vi "HFRR ADV v032 new software.vi"() -> ()   [LabVIEW 2025] (continued)
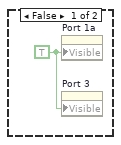
[diagram p5: hidden frame]
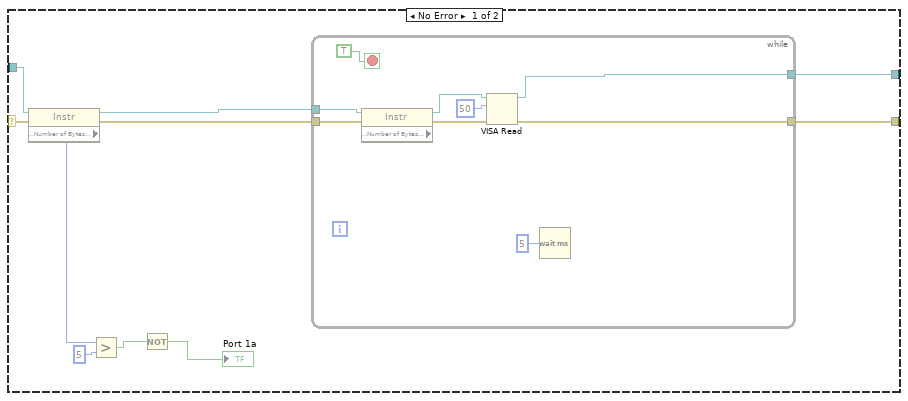
[diagram p6: hidden frame]
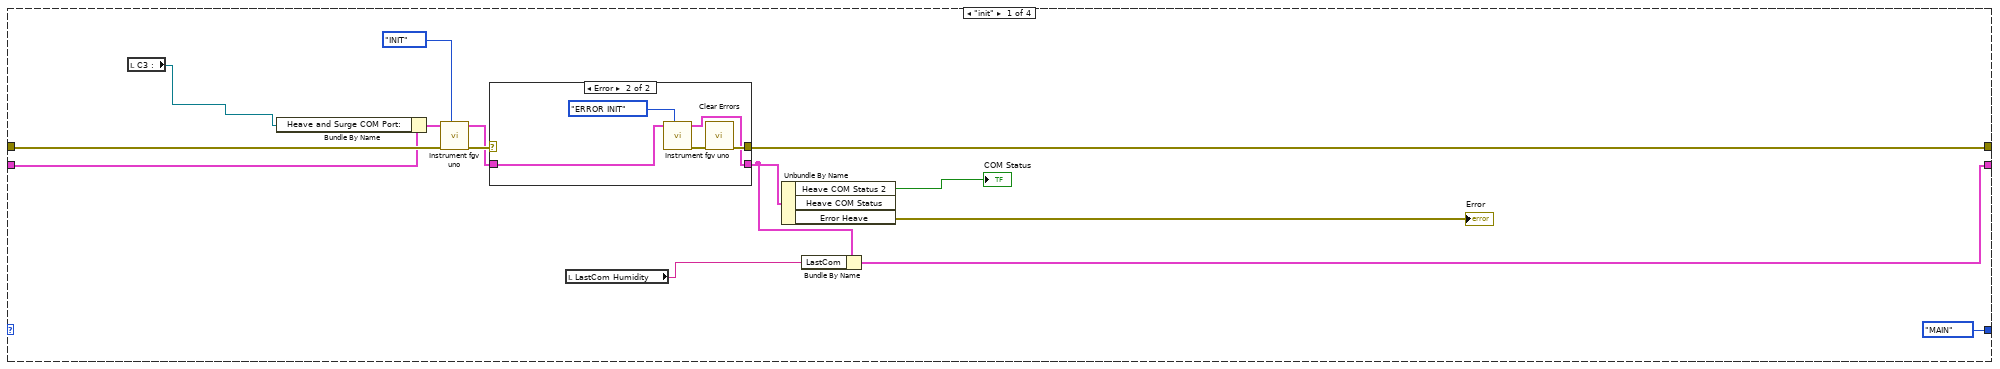
[diagram p8: hidden frame]
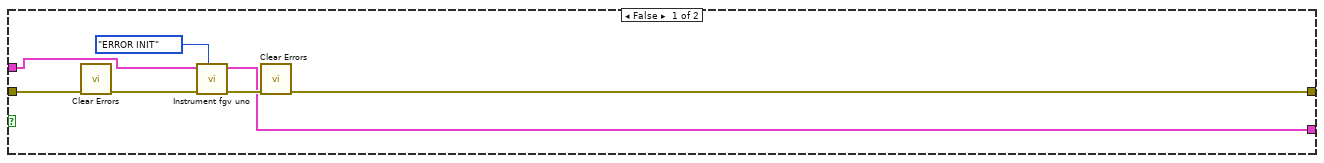
[diagram p10: hidden frame]
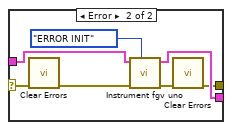
[diagram p12: hidden frame]
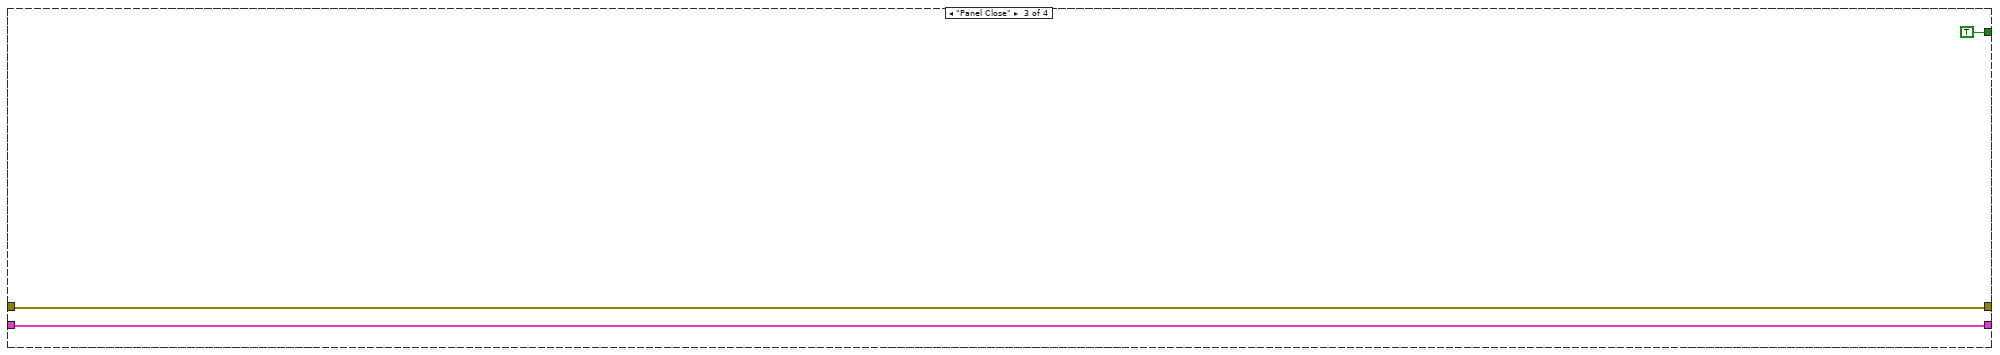
[diagram p14: hidden frame]
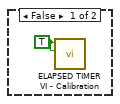
[diagram p18: hidden frame]
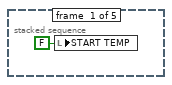
[diagram p20: hidden frame]
    shift-left: T20 {"Read Uno"="", "Bytes at Heave Port"=0.0, "UNO COM Port:"="COM9", "UNO COM Port: 2"="COM7", "Residual Due"="", "UNO COM Status 2"=TRUE, "UNO COM Status"=TRUE, "Port 2"=TRUE, "Sway PPR"=6400.0, "Surge PPR"=6400.0, "Heave PPR"=6400.0, "Sway Pitch"=2.0, "Surge Pitch"=3.0, "Heave Pitch"=4.0, "Sway Pulses/mm"=320.0, "Surge Pulses/mm"=1600.0, "Heave Pulses/mm"=1600.0, "inner loop"=0.0, "Read Heave and Surge 2"="", "String 36"="", "Write S"=FALSE, "WriteCC1"=[""], "Heave COM Loop"=0, "LastCom"="", "EXIT"=FALSE, "Error Heave"={"status"=TRUE, "code"=-1073807343, "source"=""}} -> [w4388]
    shift-right: [w4386] -> _
    shift-left: enum16{"init", "MAIN", "Panel Close"}."init" -> [w4387]
    stop <- w4390 stop-if-true
    # "UNO CODE LOGIC"
    n3353 = case shown="\"MAIN\"" w4387 {
      tunnel: w4392 -> [w4406 w4425 w4481 w4483]
      tunnel: [w4401 w4430 w4481 w4483] -> w4391
      tunnel: [_ _ TRUE _] -> w4390
      tunnel: [w4397 w4428 w4479 w4482] -> w4389
      tunnel: w4388 -> [w4403 w4424 w4479 w4482]
      tunnel: [enum16{"init", "MAIN", "Panel Close"}."MAIN" w4419 _ _] -> w4386
      frame "init" {
        n3354 = local read "Com Port 1"() -> (w4393:refnum<visa-resource-name>)
        n3355 = Bundle By Name(cluster=w4403, "UNO COM Port:"=w4393) -> (w4402:T20)
        n3356 = call "Instrument fgv.vi"("Enum"=T31."INIT", "error in (no error) 2"=w4406, "INPUT"=w4402) -> ("error"=w4404:errorcluster, "output"=w4400:T18)  [unwired: 6 in, 1 out]
        n3357 = case shown="Error" w4404 {
          selector: w4404 -> [w4408 _]
          tunnel: [w4408 w4412] -> w4401
          tunnel: w4400 -> [w4407 w4410]
          tunnel: [w4407 w4409] -> w4398
          frame No Error {
          }
          frame Error {
            n3358 = call "Instrument fgv.vi"("Enum"=T31."ERROR INIT", "INPUT"=w4410) -> ("error"=w4413:errorcluster, "output"=w4409:T18)  [unwired: 7 in, 1 out]
            n3359 = call <vilib>:"Clear Errors.vi"("error in (no error)"=w4413) -> ("error out"=w4412:errorcluster)  [unwired: 5 in, 1 out]
          }
        }
        n3360 = local read "LastCom UNO"() -> (w4395:string)
        n3361 = Unbundle By Name(w4398) -> ("Heave COM Status 2"=→"Instrument Status":bool, "Error Heave"=→"Error  2":errorcluster)  [unwired: 1 out]
        n3362 = Bundle By Name(cluster=w4398, "LastCom"=w4395) -> (w4397:T18)
      }
      frame "MAIN" {
        n3363 = Unbundle By Name(w4424) -> ("UNO COM Port: 2"=w4414:refnum<visa-resource-name>)
        n3364 = local read "Com Port 1"() -> (w4415:refnum<visa-resource-name>)
        n3365 = local write "COM Port UNO :"(w4414) -> ()
        n3366 = Equal?(x=w4414, y=w4415) -> (x = y?=w4431:bool)
        n3367 = Bundle By Name(cluster=w4424, "UNO COM Port:"=w4415) -> (w4423:T20)
        n3368 = case shown="True" w4431 {
          tunnel: [w4435 w4452] -> w4430
          tunnel: w4425 -> [w4436 w4458]
          tunnel: w4423 -> [w4434 w4456]
          tunnel: [w4433 w4451] -> w4428
          frame False {
            n3369 = call <vilib>:"Clear Errors.vi"("error in (no error)"=w4436) -> ("error out"=w4432:errorcluster)  [unwired: 5 in, 1 out]
            n3370 = call "Instrument fgv.vi"("Enum"=T31."ERROR INIT", "error in (no error) 2"=w4432, "INPUT"=w4434) -> ("error"=w4438:errorcluster, "output"=w4433:T18)  [unwired: 6 in, 1 out]
            n3371 = call <vilib>:"Clear Errors.vi"("error in (no error)"=w4438) -> ("error out"=w4435:errorcluster)  [unwired: 5 in, 1 out]
          }
          frame True {
            n3372 = call "Instrument fgv.vi"("Enum"=T31."READ", "error in (no error) 2"=w4458, "INPUT"=w4456) -> ("error"=w4457:errorcluster, "output"=w4450:T18)  [unwired: 6 in, 1 out]
            n3373 = Bundle By Name(cluster=w4450, "String 36"="WRITE UNO") -> (w4449:T18)
            n3374 = case shown="True" "Write" {
              selector: "Write" -> [_ w4473]
              tunnel: w4457 -> [w4471 w4478]
              tunnel: [w4471 w4477] -> w4447
              tunnel: w4449 -> [w4470 w4475]
              tunnel: [w4470 w4474] -> w4446
              frame False {
              }
              frame True {
                n3375 = Not(x=w4473) -> (.not. x?=w4472:bool)
                n3376 = local write "Write"(w4472) -> ()
                n3377 = call "Instrument fgv.vi"("Enum"=T31."MANUAL WRITE", "error in (no error) 2"=w4478, "INPUT"=w4475) -> ("error"=w4477:errorcluster, "output"=w4474:T18)  [unwired: 6 in, 1 out]
              }
            }
            n3378 = Array Size(array="Write UNO") -> (size(s)=w4444:i32)
            n3379 = Greater Than 0?(x=w4444) -> (x > 0?=w4443:bool)
            n3380 = call "Instrument fgv.vi"("Enum"=T31."WRITE", "error in (no error) 2"=w4447, "WriteCC1"="Write UNO", "INPUT"=w4446) -> ("error"=w4454:errorcluster, "WriteCC1 2"=w4445:string[], "output"=w4453:T18)  [unwired: 5 in]
            n3381 = case shown="True" w4443 {
              tunnel: w4445 -> [_ w4460]
              frame False {
              }
              frame True {
                n3382 = local write "Write UNO"(w4460) -> ()
              }
            }
            n3383 = case shown="Error" w4454 {
              selector: w4454 -> [w4461 w4464]
              tunnel: w4453 -> [w4462 w4469]
              tunnel: [w4462 w4468] -> w4451
              tunnel: [w4461 w4466] -> w4452
              frame No Error {
              }
              frame Error {
                n3384 = call <vilib>:"Clear Errors.vi"("error in (no error)"=w4464) -> ("error out"=w4463:errorcluster)  [unwired: 5 in, 1 out]
                n3385 = call "Instrument fgv.vi"("Enum"=T31."ERROR INIT", "error in (no error) 2"=w4463, "INPUT"=w4469) -> ("error"=w4467:errorcluster, "output"=w4468:T18)  [unwired: 6 in, 1 out]
                n3386 = call <vilib>:"Clear Errors.vi"("error in (no error)"=w4467) -> ("error out"=w4466:errorcluster)  [unwired: 5 in, 1 out]
              }
            }
            n3387 = Unbundle By Name(w4451) -> ("LastCom"=→"LastCom UNO":string, "Read Heave and Surge"=→"Read UNO":string)
          }
        }
        n3388 = Unbundle By Name(w4428) -> ("Heave COM Status 2"=w4429:bool, "Heave COM Status"=w4418:bool, "Error Heave"=w4416:errorcluster, "Bytes at Heave Port"=→"Bytes at Humidity Port":dbl)
        n3389 = Not(x=w4418) -> (.not. x?=w4426:bool)
        n3390 = Not(x=w4429) -> (.not. x?=w4417:bool)
        n3391 = local write "Instrument Status"(w4426) -> ()
        n3392 = local write "Error  2"(w4416) -> ()
        n3393 = local write "Port 1a"(w4418) -> ()
        n3394 = local read "Quit"() -> (w4420:bool)
        n3395 = local write "COM Status"(w4417) -> ()
        n3396 = Select(t=enum16{"init", "MAIN", "Panel Close"}."Panel Close", s=w4420, f=enum16{"init", "MAIN", "Panel Close"}."MAIN") -> (s? t:f=w4419:enum16{"init", "MAIN", "Panel Close"})
      }
      frame "Panel Close" {
      }
      frame Default {
      }
    }
  }
  n3397 = while {
    stop <- w4509 stop-if-true
    n3398 = local read "Read HUMIDITY"() -> (w4484:string)
    n3399 = call <vilib>:"High Resolution Polling Wait.vi"("seconds to wait"=0.05) -> ()  [unwired: 10 in, 1 out]
    n3400 = Spreadsheet String To Array(delimiter (Tab)=",", format string="", spreadsheet string=w4484, array type (2D Dbl)=string[] []) -> (array=w4504:string[])
    n3401 = for {
      tunnel: w4504 -> [w4514] mode=indexing
      tunnel: string[] ["STATE;", "SET;", "RH;", "T;", "AMB_RH;", "AMB_T;", "PUMP;", "FAN_IN;", "FAN_OUT;", "DEHUM;", "CURRENT;", "STALL;"] -> [w4513] mode=indexing
      tunnel: [w4512] -> w4503 mode=indexing
      n3402 = Match Pattern(string=w4514, regular expression=w4513) -> (after substring=w4512:string)  [unwired: 1 in, 3 out]
    }
    n3403 = Index Array(array=w4503) -> (element #1=→"STATE :":string, element #2=→"SET :":string, element #3=w4492:string, element #4=→"T :":string, element #5=w4490:string, element #6=→"AMB_T :":string, element #7=→"PUMP :":string, element #8=→"FAN_IN :":string, element #9=→"FAN_OUT :":string, element #10=→"DEHUM :":string, element #11=→"CURRENT :":string, element #12=→"STALL :":string)  [unwired: 12 in]
    "RH :" <- w4492
    "AMB_RH :" <- w4490
    n3404 = Fract/Exp String To Number(string=w4492) -> (number=w4485:dbl)  [unwired: 3 in, 1 out]
    n3405 = Fract/Exp String To Number(string=w4490) -> (number=w4489:dbl)  [unwired: 3 in, 1 out]
    n3406 = local write "Ambient Humidity :"(w4489) -> ()
    n3407 = Equal?(x=w4485, y=0.0) -> (x = y?=w4487:bool)
    n3408 = case shown="True" w4487 {
      tunnel: [w4510 w4511] -> w4486
      tunnel: w4485 -> [w4510 _]
      frame False {
        (unwired) 0.0
        "Humidity temp" <- w4510
      }
      frame True {
        n3409 = local read "Humidity temp"() -> (w4511:dbl)
      }
    }
    "RH Numeric:" <- w4486
    n3410 = local read "Quit"() -> (w4509:bool)
  }
